vi "New buffers.vi"(10 "data rate (hz)":dbl format="%#_13g", 11 "buffer (minutes)":dbl format="%#_13g") -> (2 "period (ms)":i32, 3 "ChannelMap":map{T1, refnum<data-value>}(c390))   [LabVIEW 2021, in "BluePlotDemo.lvlib"]
uses:
  BluePlotDemo.lvlib
  Demo Names.ctl
  <vilib>/National Instruments/Variant Ring Buffer/Ring Buffer.lvclass
  ring buffer data.ctl
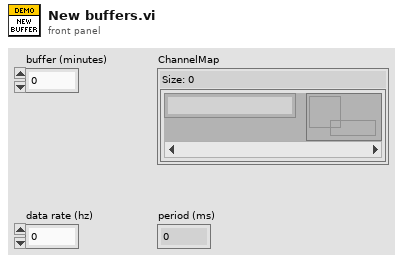
[diagram p1: front panel]
types:
  T1 = typedef "BluePlotDemo.lvlib/Demo Names.ctl" = enum16{"Sine Wave", "Triangle Wave", "Sawtooth Wave", "Square Wave", "Uniform Noise", "Periodic Noise", "White Noise"}
  T2 = typedef "BluePlotDemo.lvlib/ring buffer data.ctl" = cluster{"timestamp":dbl, "value":dbl}
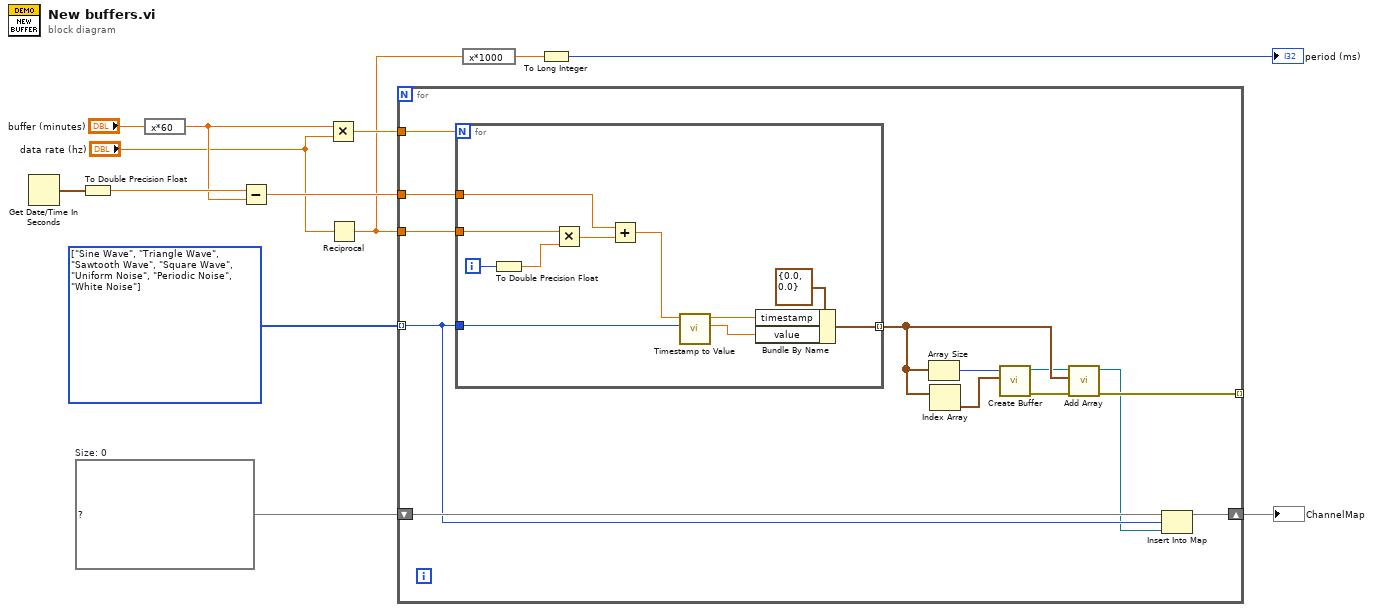
[diagram p0: block diagram]
diagram:
  w2 = map{T1, refnum<data-value>} {}  # Size: 0
  w6 = T1[] [enum."Sine Wave", enum."Triangle Wave", enum."Sawtooth Wave", enum."Square Wave", enum."Uniform Noise", enum."Periodic Noise", enum."White Noise"] items=["Sine Wave", "Triangle Wave", "Sawtooth Wave", "Square Wave", "Uniform Noise", "Periodic Noise", "White Noise"]
  n1 = Get Date/Time In Seconds() -> (seconds since 1Jan1904=w13:timestamp)
  n2 = To Double Precision Float(number=w13) -> (double precision float=w11:dbl)
  n3 = expression code="x*60"("buffer (minutes)") -> (w10:dbl)
  n4 = Subtract(x=w11, y=w10) -> (x-y=w8:dbl)
  n5 = Multiply(x=w10, y="data rate (hz)") -> (x*y=w9:dbl)
  n6 = Reciprocal(x="data rate (hz)") -> (1/x=w5:dbl)
  n7 = for {
    tunnel: w9 -> [w26]
    tunnel: w8 -> [w16]
    tunnel: w5 -> [w25]
    tunnel: w6 -> [w18] mode=indexing
    tunnel: [w21] -> _ mode=indexing
    shift-right: [w19] -> w1
    shift-left: w2 -> [w20]
    n8 = for {
      N: w26 -> [_]
      tunnel: w25 -> [w37]
      tunnel: [w31] -> w23 mode=indexing
      tunnel: w18 -> [w30]
      tunnel: w16 -> [w28]
      i -> [w36]
      n9 = To Double Precision Float(number=w36) -> (double precision float=w35:dbl)
      n10 = Multiply(x=w37, y=w35) -> (x*y=w34:dbl)
      n11 = Add(x=w28, y=w34) -> (x+y=w27:dbl)
      n12 = call "Timestamp to Value.vi"("Channel"=w30, "timestamp"=w27) -> ("value"=w32:dbl, "timestamp (dup)"=w29:dbl)  [unwired: 8 in]
      n13 = Bundle By Name(cluster=T2 {"timestamp"=0.0, "value"=0.0} ("Cluster"), "timestamp"=w29, "value"=w32) -> (w31:T2)
    }
    n14 = Array Size(array=w23) -> (size(s)=w22:i32)
    n15 = Index Array(array=w23) -> (element=w24:T2)  [unwired: 1 in]
    n16 = call <vilib>:"Create Buffer.vi"("Data Type"=w24, "Buffer Size"=w22) -> ("Error In"=w14:errorcluster, "Ring Buffer Reference"=w15:refnum<data-value>)  [unwired: 8 in]
    n17 = call <vilib>:"Add Array.vi"("Error In"=w14, "Variants Array"=w23, "Ring Buffer Reference"=w15) -> ("Error Out"=w21:errorcluster, "Ring Buffer Reference"=w17:refnum<data-value>)  [unwired: 7 in]
    n18 = Insert Into Map(map in=w20, key=w18, value=w17) -> (map out=w19:map{T1, refnum<data-value>})  [unwired: 2 out]
  }
  "ChannelMap" <- w1
  n19 = expression code="x*1000"(w5) -> (w4:dbl)
  n20 = To Long Integer(number=w4) -> (32bit integer=→"period (ms)":i32)
